vi "SIM_CurrentOutput.vi"(9 "array":dbl[][](array[numeric]), 10 "Position (Reframed)":cluster{"x (m)":dbl, "y (m)":dbl, "z (mm)":dbl} {"z (mm)" format="%.1f"; "y (m)" format="%.1p"; "x (m)" format="%.1p"}, 11 "Current Mode":bool=TRUE) -> (3 "Signal Out":dbl, 4 "Zread":dbl, 6 "z (mm)":dbl)   [LabVIEW 2022 SP3]
uses:
  <vilib>/ptbypt/NI_PtbyPt.lvlib
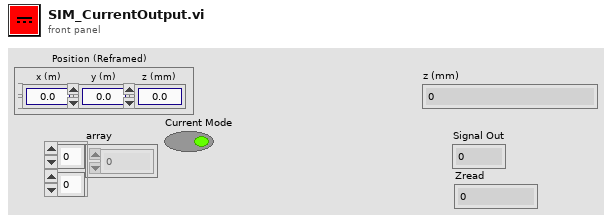
[diagram p1: front panel]
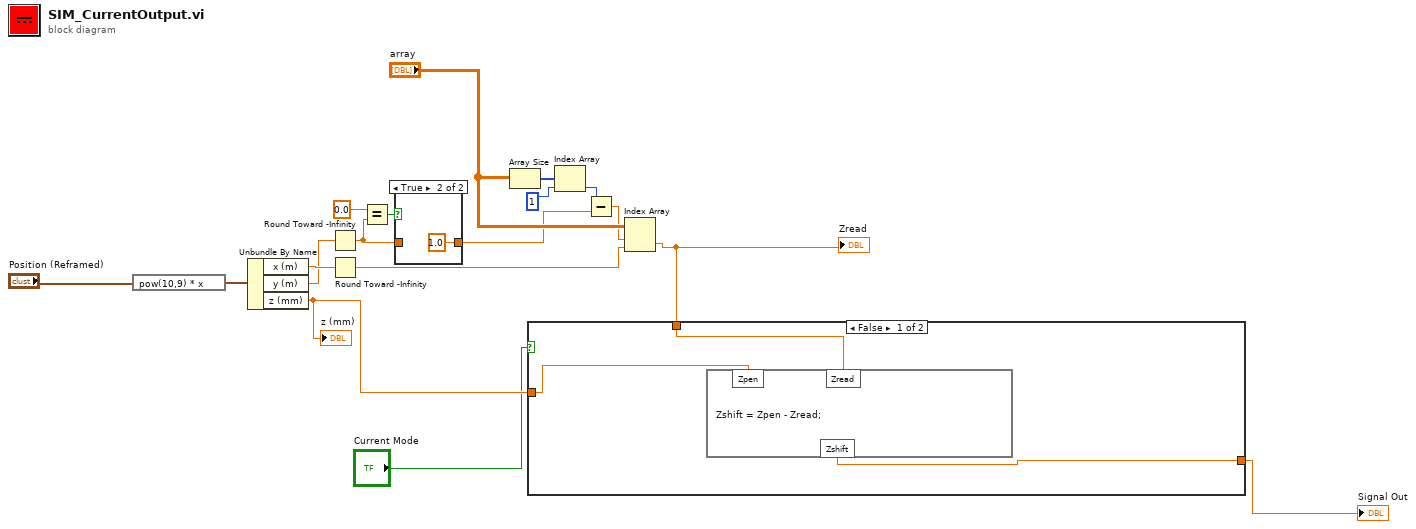
[diagram p0: block diagram]
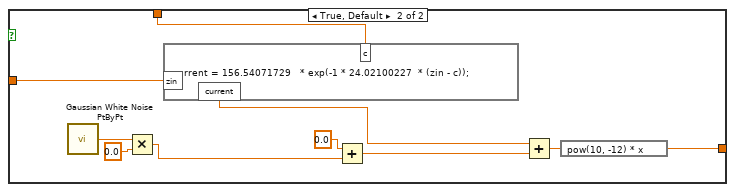
[diagram p2: hidden frame]
diagram:
  n1 = expression code="pow(10,9) * x"("Position (Reframed)") -> (w16:cluster{"x (m)":dbl, "y (m)":dbl, "z (mm)":dbl})
  n2 = Unbundle By Name(w16) -> ("x (m)"=w15:dbl, "y (m)"=w14:dbl, "z (mm)"=w3:dbl)
  "z (mm)" <- w3
  n3 = Round Toward -Infinity(1:w14) -> (0:w5:dbl)
  n4 = Round Toward -Infinity(1:w15) -> (0:w18:dbl)
  n5 = Equal?(x=0.0, y=w5) -> (x = y?=w8:bool)
  n6 = case shown="True" w8 {
    tunnel: [w19 1.0] -> w6
    tunnel: w5 -> [w19 _]
    frame False {
    }
    frame True {
    }
  }
  n7 = Array Size(array="array") -> (size(s)=w12:i32[])
  n8 = Index Array(array=w12, index=1) -> (element=w9:i32)
  n9 = Subtract(x=w9, y=w6) -> (x-y=w10:dbl)
  n10 = Index Array(array="array", index (row)=w10, index (col)=w18) -> (element=w4:dbl)
  "Zread" <- w4
  n11 = case shown="False" "Current Mode" {
    tunnel: w4 -> [w22 w33]
    tunnel: w3 -> [w23 w32]
    tunnel: [w21 w24] -> w1
    frame False {
      n12 = formula code="Zshift = Zpen - Zread;"("Zread"=w22, "Zpen"=w23) -> ("Zshift"=w21:dbl)
    }
    frame True, Default {
      n13 = call <vilib>:"Gaussian White Noise PtByPt.vi"() -> ("Gaussian white noise"=w30:dbl)  [unwired: 3 in]
      n14 = Multiply(x=w30, y=0.0) -> (x*y=w26:dbl)
      n15 = formula code="current = 156.54071729   * exp(-1 * 24.02100227  * (zin - c));"("zin"=w32, "c"=w33) -> ("current"=w27:dbl)
      n16 = Add(x=0.0, y=w26) -> (x+y=w31:dbl)
      n17 = Add(x=w27, y=w31) -> (x+y=w25:dbl)
      n18 = expression code="pow(10, -12) * x"(w25) -> (w24:dbl)
    }
  }
  "Signal Out" <- w1
